vi "Global_SM_Output.vi"() -> ()   [LabVIEW 2017]
uses:
  ENUM_Rotation_Positon.ctl
  Rotation_Overlord.lvlib
panel:
  in  "SM_Rotation_Output":T1=enum."Manual"
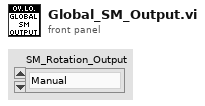
[diagram p1: front panel]
types:
  T1 = typedef "Rotation_Overlord.lvlib/ENUM_Rotation_Positon.ctl" = enum16{"Neutral", "Pickup", "Switch", "Scale", "Climb", "Manual"}
diagram:
